vi "Spartan HTTP Parse Request.vi"(8 "error in (no error)":errorcluster, 9 "Content-length (-1)":i32=-1, 10 "HTTP Request (\"\")":string, 11 "HTTP Data":T1 {"object data"."time" format="%0.2f"}) -> (0 "error out":errorcluster, 3 "dup http session":T1 {"object data"."time" format="%0.2f"})   [LabVIEW 2011]
uses:
  Spartan HTTP Session.ctl
  ITK EXT/http/http_obj.llb/HTTP Session Data.ctl
  ITK EXT/utils/keyedarr.llb/Keyed Array.ctl
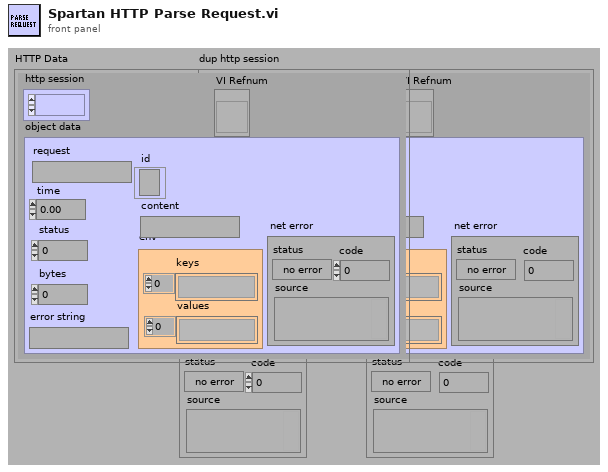
[diagram p1: front panel]
types:
  T1 = typedef "Spartan HTTP Session.ctl" = cluster{"http session":refnum<k1>, "object data":T2, "VI Refnum":refnum<vi>}
  T2 = typedef "HTTP Session Data.ctl" = cluster{"request":string, "time":dbl, "status":i32, "error string":string, "bytes":i32, "env":T3, "content":string, "id":refnum<k5>, "net error":errorcluster}
  T3 = typedef "Keyed Array.ctl" = cluster{"keys":string[], "values":string[]}
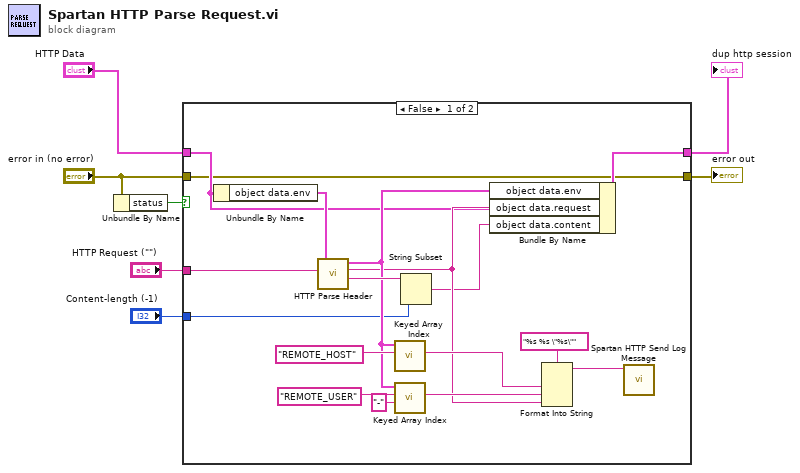
[diagram p0: block diagram]
diagram:
  n1 = Unbundle By Name("error in (no error)") -> ("status"=w7:bool)
  n2 = case shown="False" w7 {
    tunnel: "error in (no error)" -> [w8 w26]
    tunnel: [w8 w26] -> w5
    tunnel: "HTTP Data" -> [w10 w25]
    tunnel: "HTTP Request (\"\")" -> [w12 _]
    tunnel: "Content-length (-1)" -> [w11 _]
    tunnel: [w9 w25] -> w1
    frame False {
      n3 = Unbundle By Name(w10) -> ("object data.env"=w24:T3)
      n4 = call "HTTP Parse Header.vi"("server message"=w12, "env"=w24) -> ("content"=w23:string, "request"=w14:string, "env out"=w18:T3)  [unwired: 3 out]
      n5 = call "Keyed Array Index.vi"("key"="REMOTE_HOST", "array in"=w18) -> ("value"=w20:string)  [unwired: 2 in, 3 out]
      n6 = call "Keyed Array Index.vi"("default value"="-", "key"="REMOTE_USER", "array in"=w18) -> ("value"=w16:string)  [unwired: 1 in, 3 out]
      n7 = String Subset(string=w23, length (rest)=w11) -> (substring=w13:string)  [unwired: 1 out]
      n8 = Bundle By Name(cluster=w10, "object data.env"=w18, "object data.request"=w14, "object data.content"=w13) -> (w9:T1)
      n9 = Format Into String(format string="%s %s \"%s\"", w20, w16, w14) -> (resulting string=w15:string)  [unwired: 2 in, 1 out]
      n10 = call "Spartan HTTP Send Log Message.vi"("message"=w15) -> ()  [unwired: 7 out]
    }
    frame True {
    }
  }
  "error out" <- w5
  "dup http session" <- w1
